vi "Load Template.vi"(8 "error in (no error)":errorcluster, 10 "VisionProjectName":string[](array[string]), 11 "root":path) -> (0 "error out":errorcluster)   [LabVIEW 2019]
uses:
  iVision/Analysis/Controls/Analysis_Setting.ctl
  iVision/Analysis/Controls/V_Analysis_Type.ctl
  f9af3691-598d-40a7-a07e-1061da3c4e6c.vi
  3627a59a-e9cb-4654-bdca-c49a8f8e7788.vi
  <vilib>/JDP Science/JSONtext/JSON text to Variant.vi
panel:
  out "Image":T1(plugin-control)
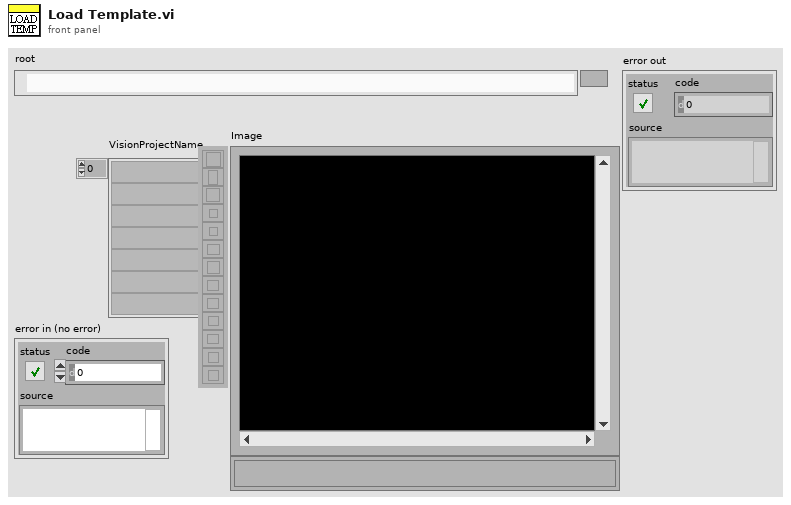
[diagram p1: front panel]
types:
  T1 = typedef "IMAQ Image.ctl" = refnum<image>
  T2 = enum16{"initial", "write", "add", "delete", "Load", "Save", "Read", "ReadProjectName"}
  T3 = typedef "Analysis_Setting.ctl" = cluster{"PreProcess":T4, "Parameter":string}
  T4 = typedef "V_Analysis_Type.ctl" = enum16{"None", "C_Color Pattern Matching", "G_PatternMatching", "G_ShapeDectect", "G_GeometricMatch", "B_Area Check"}
  T5 = cluster{"ProjectName":string, "Parameter":string[][]}
  T6 = typedef "Image Type" = u32
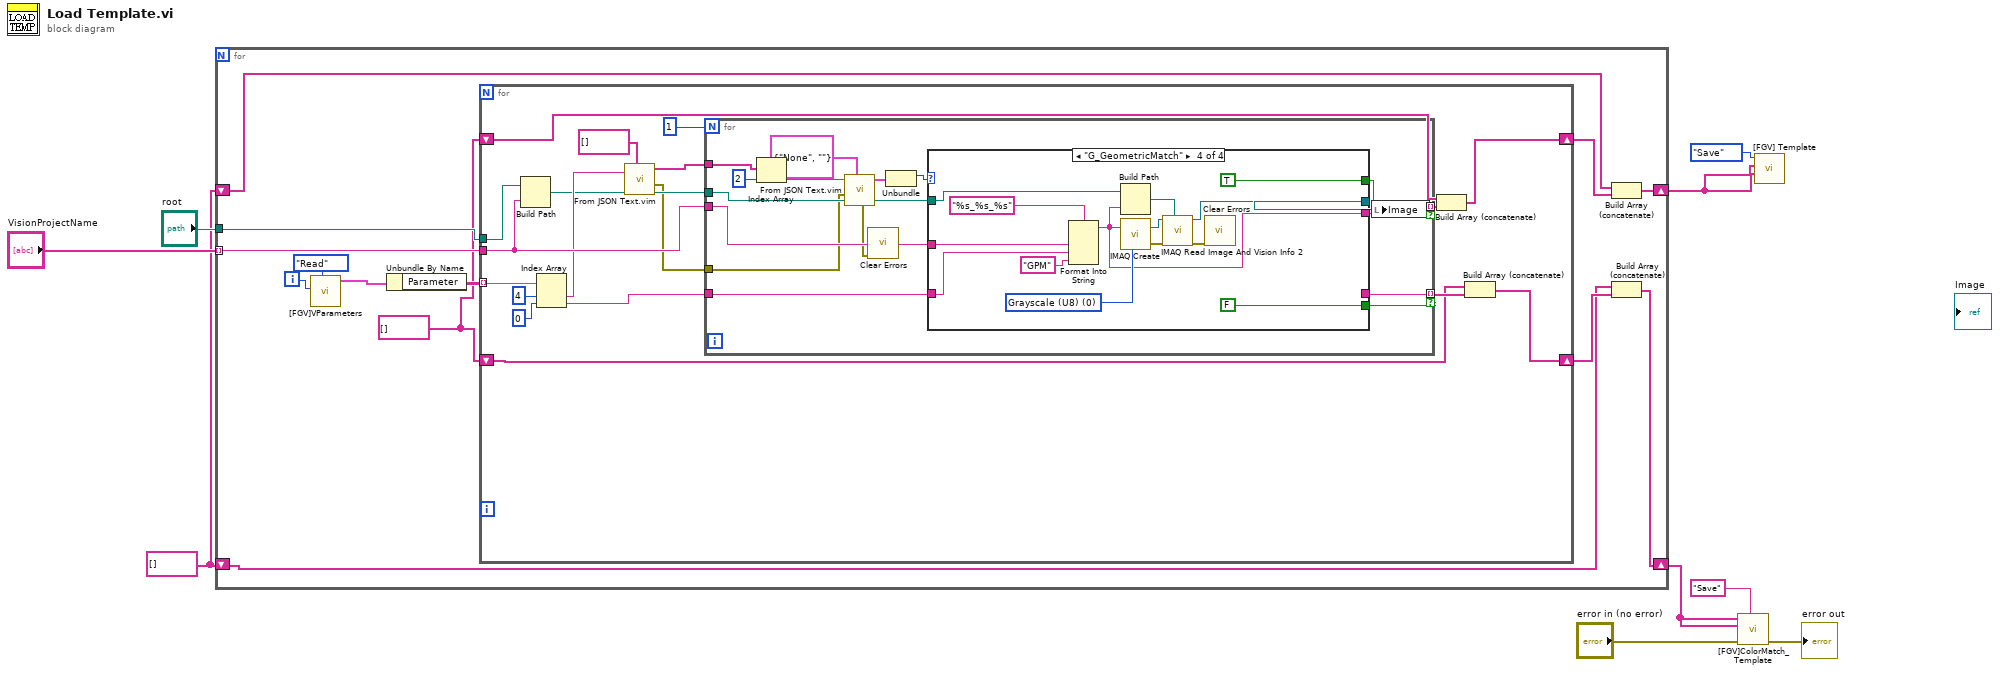
[diagram p0: block diagram]
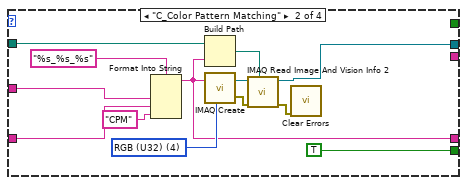
[diagram p3: hidden frame]
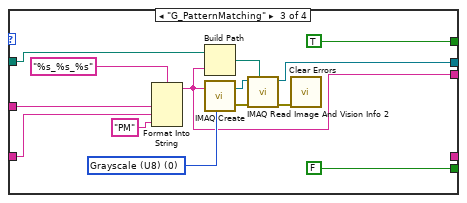
[diagram p4: hidden frame]
diagram:
  w3 = string[] []
  n1 = for {
    tunnel: "VisionProjectName" -> [w21] mode=indexing
    tunnel: "root" -> [w22]
    shift-right: [w16] -> w2
    shift-left: w3 -> [w15]
    shift-right: [w13] -> w1
    shift-left: w3 -> [w12]
    i -> [w18]
    w11 = string[] []
    n2 = call "[FGV]VParameters.vi"("Enum"=T2."Read", "ProjectIndex"=w18) -> ("DataOut"=w19:T5)  [unwired: 6 in, 3 out]
    n3 = Unbundle By Name(w19) -> ("Parameter"=w17:string[][])
    n4 = for {
      tunnel: w22 -> [w35]
      tunnel: w17 -> [w33] mode=indexing
      tunnel: w21 -> [w34]
      shift-right: [w30] -> w14
      shift-left: w11 -> [w29]
      shift-right: [w27] -> w10
      shift-left: w11 -> [w28]
      n5 = Build Path(base path=w35, name or relative path=w34) -> (appended path=w25:path)
      n6 = Index Array(array=w33, index #1=4 ("index"), index #2=0 ("index")) -> (element #1=w32:string, element #2=w38:string)
      n7 = call "From JSON Text.vim"("Data Type and Default Value"=string[] [], "JSON"=w32) -> ("error out"=w23:errorcluster, "Data out"=w26:string[])  [unwired: 8 in]
      n8 = for {
        N: 1 -> [_]
        tunnel: w25 -> [w49]
        tunnel: w38 -> [w53]
        tunnel: [w52] -> w37 mode=indexing if=w45
        tunnel: w34 -> [w50]
        tunnel: [w51] -> w36 mode=indexing if=w46
        tunnel: w26 -> [w44]
        tunnel: w23 -> [w41]
        n9 = Index Array(array=w44, index=2 ("disabled index (col)")) -> (element=w48:string)
        n10 = call "From JSON Text.vim"("Data Type and Default Value"=T3 {"PreProcess"=enum."None", "Parameter"=""} ("Analysis_Setting In"), "error in (no error)"=w41, "JSON"=w48) -> ("error out"=w42:errorcluster, "Data out"=w55:T3)  [unwired: 7 in]
        n11 = call <vilib>:"Clear Errors.vi"("error in (no error)"=w42) -> ()  [unwired: 5 in, 2 out]
        n12 = Unbundle(w55) -> ("PreProcess"=w54:T4)  [unwired: 1 out]
        n13 = case shown="\"G_GeometricMatch\"" w54 {
          tunnel: w50 -> [_ w68 w82 w96]
          tunnel: w53 -> [_ w67 w81 w95]
          tunnel: w49 -> [_ w60 w74 w88]
          tunnel: [_ TRUE FALSE FALSE] -> w45
          tunnel: [_ w58 _ _] -> w52
          tunnel: [_ _ TRUE TRUE] -> w46
          tunnel: [_ _ w71 w85] -> w51
          tunnel: [_ w57 w70 w84] -> w43
          frame Default {
          }
          frame "C_Color Pattern Matching" {
            w63 = T6 4 items=["Grayscale (U8)", "Grayscale (I16)", "Grayscale (SGL)", "Complex (CSG)", "RGB (U32)", "HSL (U32)", "RGB (U64)", "Grayscale (U16)"] ("Image Type")
            n14 = Format Into String(format string="%s_%s_%s", w68, w67, "CPM" ("input 3")) -> (resulting string=w58:string)  [unwired: 2 in, 1 out]
            n15 = Build Path(base path=w60, name or relative path=w58) -> (appended path=w64:path)
            n16 = call "IMAQ Create"("Image Name"=w58, "Image Type"=w63) -> ("New Image"=w65:T1, "error out"=w62:errorcluster)  [unwired: 3 in]
            n17 = call "IMAQ Read Image And Vision Info 2"("File Path"=w64, "error in (no error)"=w62, "Image"=w65) -> ("error out"=w61:errorcluster, "Image Out"=w57:T1)  [unwired: 6 in, 1 out]
            n18 = call <vilib>:"Clear Errors.vi"("error in (no error)"=w61) -> ()  [unwired: 5 in, 2 out]
          }
          frame "G_PatternMatching" {
            w77 = T6 0 items=["Grayscale (U8)", "Grayscale (I16)", "Grayscale (SGL)", "Complex (CSG)", "RGB (U32)", "HSL (U32)", "RGB (U64)", "Grayscale (U16)"] ("Image Type")
            n19 = Format Into String(format string="%s_%s_%s", w82, w81, "PM" ("input 3")) -> (resulting string=w71:string)  [unwired: 2 in, 1 out]
            n20 = Build Path(base path=w74, name or relative path=w71) -> (appended path=w78:path)
            n21 = call "IMAQ Create"("Image Name"=w71, "Image Type"=w77) -> ("New Image"=w79:T1, "error out"=w76:errorcluster)  [unwired: 3 in]
            n22 = call "IMAQ Read Image And Vision Info 2"("File Path"=w78, "error in (no error)"=w76, "Image"=w79) -> ("error out"=w75:errorcluster, "Image Out"=w70:T1)  [unwired: 6 in, 1 out]
            n23 = call <vilib>:"Clear Errors.vi"("error in (no error)"=w75) -> ()  [unwired: 5 in, 2 out]
          }
          frame "G_GeometricMatch" {
            w91 = T6 0 items=["Grayscale (U8)", "Grayscale (I16)", "Grayscale (SGL)", "Complex (CSG)", "RGB (U32)", "HSL (U32)", "RGB (U64)", "Grayscale (U16)"] ("Image Type")
            n24 = Format Into String(format string="%s_%s_%s", w96, w95, "GPM" ("input 3")) -> (resulting string=w85:string)  [unwired: 2 in, 1 out]
            n25 = Build Path(base path=w88, name or relative path=w85) -> (appended path=w92:path)
            n26 = call "IMAQ Create"("Image Name"=w85, "Image Type"=w91) -> ("New Image"=w93:T1, "error out"=w90:errorcluster)  [unwired: 3 in]
            n27 = call "IMAQ Read Image And Vision Info 2"("File Path"=w92, "error in (no error)"=w90, "Image"=w93) -> ("error out"=w89:errorcluster, "Image Out"=w84:T1)  [unwired: 6 in, 1 out]
            n28 = call <vilib>:"Clear Errors.vi"("error in (no error)"=w89) -> ()  [unwired: 5 in, 2 out]
          }
        }
        n29 = local write "Image"(w43) -> ()
      }
      n30 = Build Array (concatenate)(w28, w36) -> (w27:string[])
      n31 = Build Array (concatenate)(w29, w37) -> (w30:string[])
    }
    n32 = Build Array (concatenate)(w15, w10) -> (w16:string[])
    n33 = Build Array (concatenate)(w12, w14) -> (w13:string[])
  }
  n34 = call "[FGV]ColorMatch_Template.vi"("CMTemplateCommand"="Save", "error in (no error)"="error in (no error)", "Image Name Array"=w1, "Image Array"=w1) -> ("error out"=→"error out":errorcluster)  [unwired: 5 in, 2 out]
  n35 = call "[FGV] Template.vi"("Image Name Array"=w2, "Image Array"=w2, "Command"=enum16{"Initialize", "Save", "Read"}."Save") -> ()  [unwired: 6 in, 3 out]
